vi "VRM_DSC.vi"() -> ()   [LabVIEW 2013]
uses:
  <vilib>/Utility/file.llb/Read From Spreadsheet File (string).vi
panel:
  in  "milliseconds to wait":u32=2500
  in  "stop":bool
  # "This program reads the VRM log and write into DSC, once every"
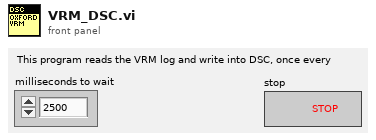
[diagram p1: front panel]
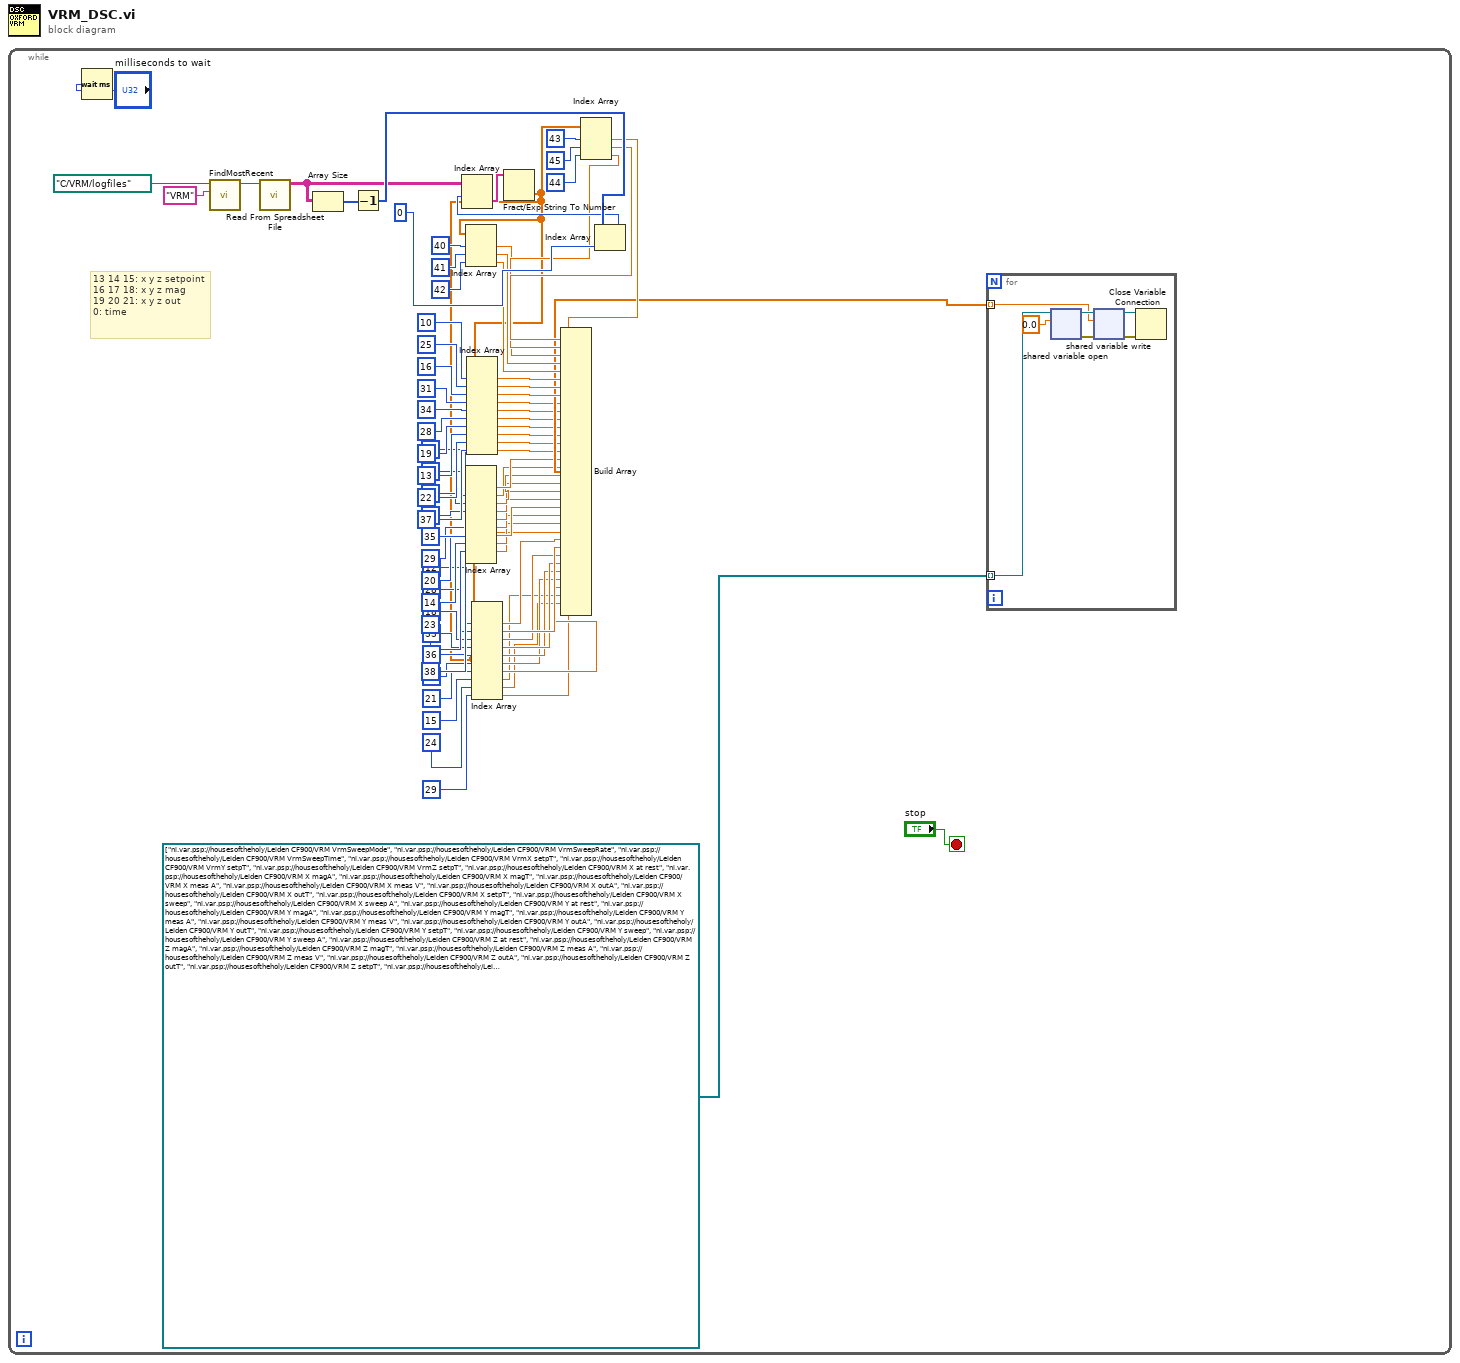
[diagram p0: block diagram]
diagram:
  n1 = while {
    stop <- "stop" stop-if-true
    # "13 14 15: x y z setpoint\n16 17 18: x y z mag\n19 20 21: x y z out\n0: time"
    n2 = Wait (ms)(milliseconds to wait="milliseconds to wait") -> ()  [unwired: 1 out]
    n3 = call "FindMostRecent.vi"("Filename Pattern"="VRM" ("Pattern to Match"), "Folder Path In"=path "C:/VRM/logfiles") -> ("File Path for the Newest File"=w85:path)  [unwired: 8 in, 1 out]
    n4 = call-poly <vilib>:"Read From Spreadsheet File.vi"("file path (dialog if empty)"=w85) -> ("all rows"=w80:string[][])  [unwired: 6 in, 4 out]
    n5 = Array Size(array=w80) -> (size(s)=w84:i32[])
    n6 = Decrement(x=w84) -> (x-1=w83:i32[])
    n7 = Index Array(array=w83, index=0) -> (element=w81:i32)
    n8 = Index Array(array=w80, index (row)=w81) -> (element=w79:string[])  [unwired: 1 in]
    n9 = Fract/Exp String To Number(string=w79) -> (number=w28:dbl[])  [unwired: 4 out]
    n10 = Index Array(array=w28, index #1=40 ("index"), index #2=41 ("index"), index #3=42 ("index")) -> (element #1=w66:dbl, element #2=w65:dbl, element #3=w64:dbl)
    n11 = Index Array(array=w28, index #1=11 ("index"), index #2=27 ("index"), index #3=17 ("index"), index #4=32 ("index"), index #5=35 ("index"), index #6=29 ("index"), index #7=20 ("index"), index #8=14 ("index"), index #9=23 ("index"), index #10=38 ("index")) -> (element #1=w20:dbl, element #2=w19:dbl, element #3=w18:dbl, element #4=w17:dbl, element #5=w16:dbl, element #6=w15:dbl, element #7=w14:dbl, element #8=w13:dbl, element #9=w12:dbl, element #10=w11:dbl)
    n12 = Index Array(array=w28, index #1=10 ("index"), index #2=25 ("index"), index #3=16 ("index"), index #4=31 ("index"), index #5=34 ("index"), index #6=28 ("index"), index #7=19 ("index"), index #8=13 ("index"), index #9=22 ("index"), index #10=37 ("index")) -> (element #1=w63:dbl, element #2=w62:dbl, element #3=w61:dbl, element #4=w27:dbl, element #5=w26:dbl, element #6=w21:dbl, element #7=w22:dbl, element #8=w23:dbl, element #9=w24:dbl, element #10=w25:dbl)
    n13 = Index Array(array=w28, index #1=12 ("index"), index #2=28 ("index"), index #3=18 ("index"), index #4=33 ("index"), index #5=36 ("index"), index #6=30 ("index"), index #7=21 ("index"), index #8=15 ("index"), index #9=24 ("index"), index #10=29 ("index")) -> (element #1=w10:dbl, element #2=w9:dbl, element #3=w8:dbl, element #4=w7:dbl, element #5=w6:dbl, element #6=w5:dbl, element #7=w4:dbl, element #8=w3:dbl, element #9=w2:dbl, element #10=w1:dbl)
    n14 = Index Array(array=w28, index #1=43 ("index"), index #2=45 ("index"), index #3=44 ("index")) -> (element #1=w69:dbl, element #2=w68:dbl, element #3=w67:dbl)
    n15 = Build Array(w69, w68, w67, w66, w65, w64, w63, w62, w61, w27, w26, w21, w22, w23, w24, w25, w20, w19, w18, w17, w16, w15, w14, w13, w12, w11, w10, w9, w8, w7, w6, w5, w4, w3, w2, w1) -> (w59:dbl[])
    n16 = for {
      tunnel: refnum<k21>[] ["ni.var.psp://housesoftheholy/Leiden CF900/VRM VrmSweepMode", "ni.var.psp://housesoftheholy/Leiden CF900/VRM VrmSweepRate", "ni.var.psp://housesoftheholy/Leiden CF900/VRM VrmSweepTime", "ni.var.psp://housesoftheholy/Leiden CF900/VRM VrmX setpT", "ni.var.psp://housesoftheholy/Leiden CF900/VRM VrmY setpT", "ni.var.psp://housesoftheholy/Leiden CF900/VRM VrmZ setpT", "ni.var.psp://housesoftheholy/Leiden CF900/VRM X at rest", "ni.var.psp://housesoftheholy/Leiden CF900/VRM X magA", "ni.var.psp://housesoftheholy/Leiden CF900/VRM X magT", "ni.var.psp://housesoftheholy/Leiden CF900/VRM X meas A", "ni.var.psp://housesoftheholy/Leiden CF900/VRM X meas V", "ni.var.psp://housesoftheholy/Leiden CF900/VRM X outA", "ni.var.psp://housesoftheholy/Leiden CF900/VRM X outT", "ni.var.psp://housesoftheholy/Leiden CF900/VRM X setpT", "ni.var.psp://housesoftheholy/Leiden CF900/VRM X sweep", "ni.var.psp://housesoftheholy/Leiden CF900/VRM X sweep A", "ni.var.psp://housesoftheholy/Leiden CF900/VRM Y at rest", "ni.var.psp://housesoftheholy/Leiden CF900/VRM Y magA", "ni.var.psp://housesoftheholy/Leiden CF900/VRM Y magT", "ni.var.psp://housesoftheholy/Leiden CF900/VRM Y meas A", "ni.var.psp://housesoftheholy/Leiden CF900/VRM Y meas V", "ni.var.psp://housesoftheholy/Leiden CF900/VRM Y outA", "ni.var.psp://housesoftheholy/Leiden CF900/VRM Y outT", "ni.var.psp://housesoftheholy/Leiden CF900/VRM Y setpT", "ni.var.psp://housesoftheholy/Leiden CF900/VRM Y sweep", "ni.var.psp://housesoftheholy/Leiden CF900/VRM Y sweep A", "ni.var.psp://housesoftheholy/Leiden CF900/VRM Z at rest", "ni.var.psp://housesoftheholy/Leiden CF900/VRM Z magA", "ni.var.psp://housesoftheholy/Leiden CF900/VRM Z magT", "ni.var.psp://housesoftheholy/Leiden CF900/VRM Z meas A", "ni.var.psp://housesoftheholy/Leiden CF900/VRM Z meas V", "ni.var.psp://housesoftheholy/Leiden CF900/VRM Z outA", "ni.var.psp://housesoftheholy/Leiden CF900/VRM Z outT", "ni.var.psp://housesoftheholy/Leiden CF900/VRM Z setpT", "ni.var.psp://housesoftheholy/Leiden CF900/VRM Z sweep", "ni.var.psp://housesoftheholy/Leiden CF900/VRM Z sweep A"] -> [w88] mode=indexing
      tunnel: w59 -> [w87] mode=indexing
      n17 = shared-variable-open(w88, 0.0) -> (w91:refnum<k21>, w90:errorcluster)  [unwired: 2 in]
      n18 = shared-variable-write(w91, w90, w87) -> (w92:refnum<k21>, w89:errorcluster)
      n19 = Close Variable Connection(8:w89, 11:w92) -> ()  [unwired: 1 out]
    }
  }
